vi "SCB-HMI.vi"() -> ()   [LabVIEW 2016]
uses:
  SC2 states.ctl
  Interface states.ctl
  Bypass control.ctl
  Minimum Times.ctl
  Vertical Rod states.ctl
  Horizontal Rod states.ctl
  GV states.ctl
panel:
  in  "Tab Control":T1(tab)
  in  "Start Rotate Wheel":bool
  in  "Wheel GV":bool
  in  "Ion Source GV":bool
  in  "Sample Rod":bool
  in  "Retract Rod":bool
  in  "Insert Rod":bool
  in  "Random Change":bool
  in  "Requested Sample":u8=32
  in  "Start Sample Change":bool
  in  "stop":bool
  out "Monitor state (CP)":T2=enum."Wait"
  out "Current Sample (CP)":u8
  out "Encoder Position":i32
  out "Converted Encoder":bool[](array[boolean])
  out "Raw Encoder":bool[](array[boolean])
  out "SCB State Control":T3=enum."wait"
  out "Current Sample":u8
  out "Change Complete?":bool
  out "Monitor State":T2=enum."Wait"
  out "Encoder Radius Readback":dbl=2.0
  out "Encoder Destination":i32
  out "Motor status":bool=TRUE
  out "Wheel GV Status":enum16{"status unclear", "closed", "open"}(ring)
  out "Insert Rod Status":enum16{"status unclear", "rod in", "rod out"}(ring)
  out "Ion Source GV Status":enum16{"status unclear", "closed", "open"}(ring)
  out "Sample Rod Status":enum16{"status unclear", "rod down", "rod up"}(ring)
  out "Retract Rod Status":enum16{"status unclear", "rod in", "rod out"}(ring)
  out "Sample Changer Status":string
  out "Requested Sample":u8
  in  "Bypass Cluster":T4
  in  "Encoder Radius":dbl=1.0
  in  "Encoder Offset":i16=-1021
  in  "Timeouts (ms)":T5={"Sample Rod"=10000, "Insert Rod"=10000, "Retract Rod"=10000, "Wheel GV"=10000, "Ion Source GV"=10000, "Rotate Wheel"=15000}
  in  "Minimum Times (ms)":T6={"Rotate Wheel Minimum Time"=1000}
  out "error out":errorcluster
  in  "error in (no error)":errorcluster
  # "Close"
  # "Open"
  # "Close"
  # "Open"
  # "Raise"
  # "Lower"
  # "Retract"
  # "Insert"
  # "Retract"
  # "Insert"
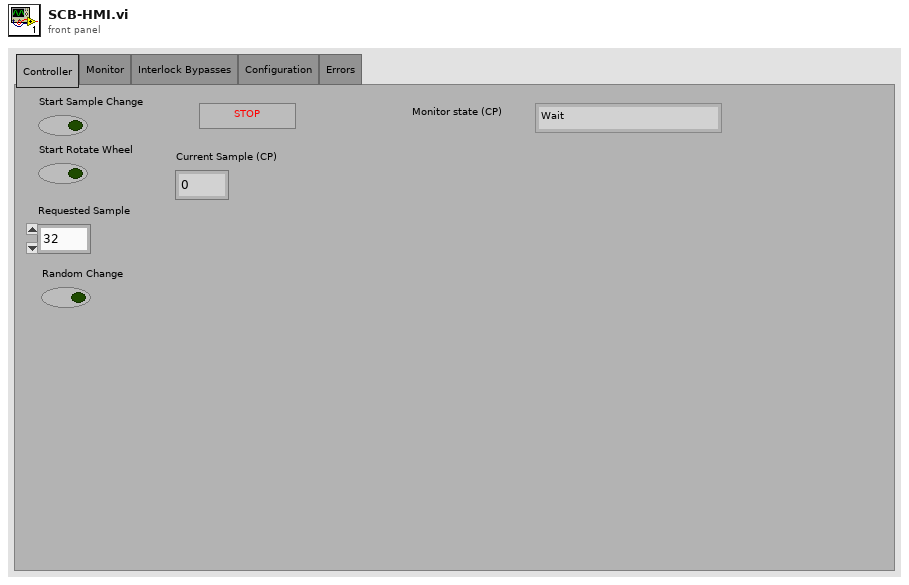
[diagram p1: front panel]
types:
  T1 = enum32{"Controller", "Monitor", "Interlock Bypasses", "Configuration", "Errors"}
  T2 = typedef "Interface states.ctl" = enum16{"Initialization", "Wait", "start wheel change", "Start Rotate Wheel", "Shutdown"}
  T3 = typedef "SC2 states.ctl" = enum16{"initialize", "wait", "change sample start", "change sample", "check position", "rotate wheel", "sample change complete", "sample rod up", "sample rod down", "retract rod in", "retract rod out", "insert rod in", "insert rod out", "wheel GV open", "wheel GV close", "ion source GV open", "ion source GV close", "vent source", "pump source", "Shutdown"}
  T4 = typedef "Bypass control.ctl" = cluster{"SCB Insert Rod Bypass":bool, "SCB Ion Source GV Bypass":bool, "SCB Retract Rod Bypass":bool, "SCB Sample Rod Bypass":bool, "SCB Wheel GV Bypass":bool}
  T5 = cluster{"Sample Rod":u16, "Insert Rod":u16, "Retract Rod":u16, "Wheel GV":u16, "Ion Source GV":u16, "Rotate Wheel":u16}
  T6 = typedef "Minimum Times.ctl" = cluster{"Rotate Wheel Minimum Time":u16}
  T7 = typedef "Horizontal Rod states.ctl" = enum16{"status unclear", "rod in", "rod out"}
  T8 = typedef "Vertical Rod states.ctl" = enum16{"status unclear", "rod down", "rod up"}
  T9 = typedef "GV states.ctl" = enum16{"status unclear", "closed", "open"}
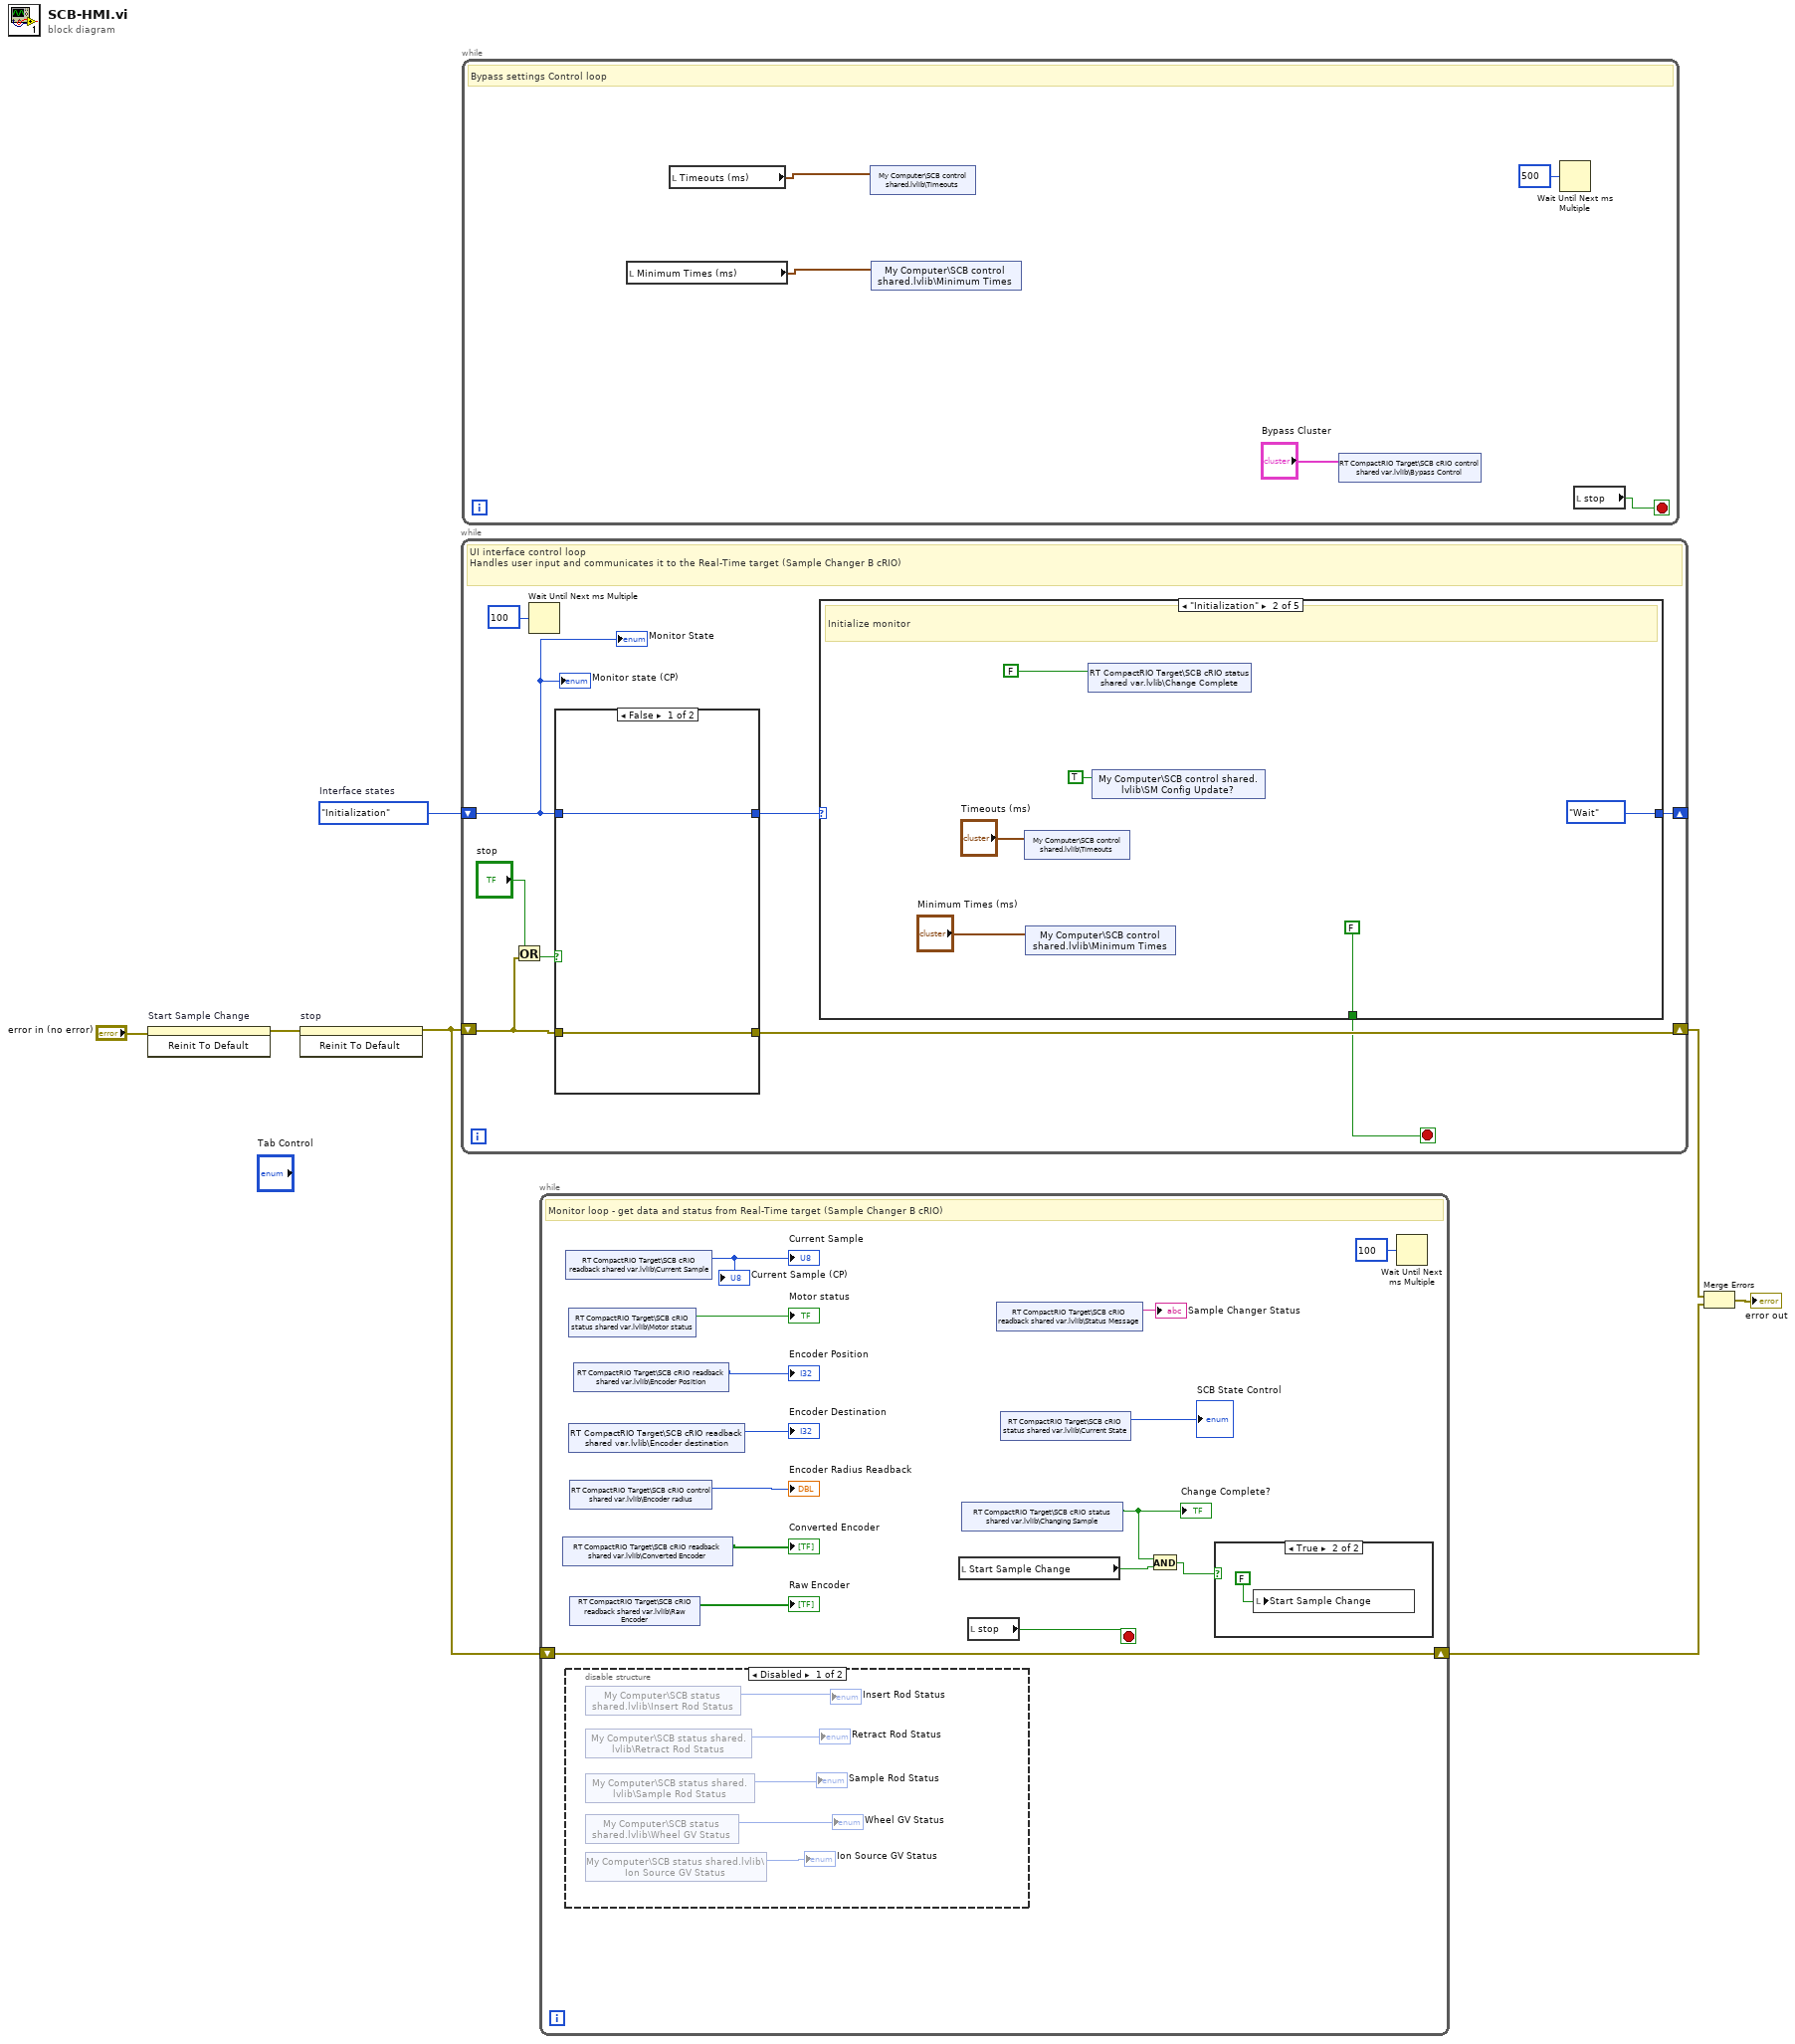
[diagram p0: block diagram]
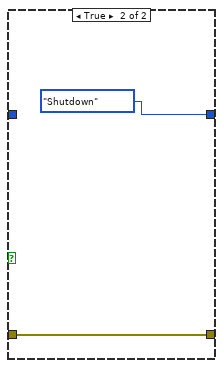
[diagram p4: hidden frame]
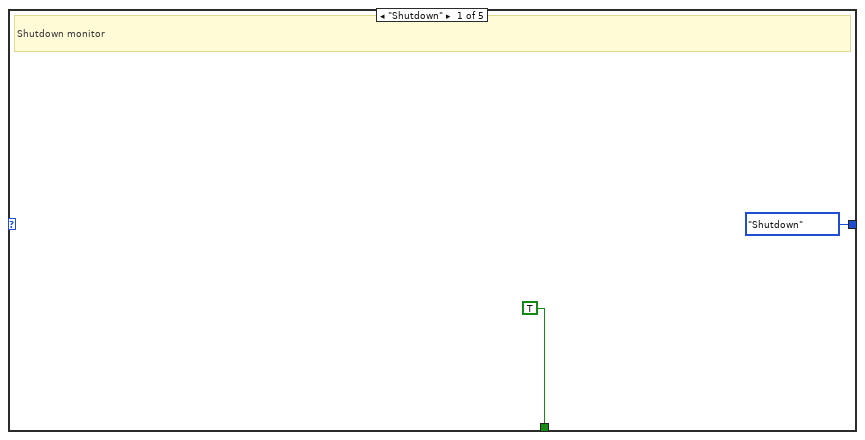
[diagram p5: hidden frame]
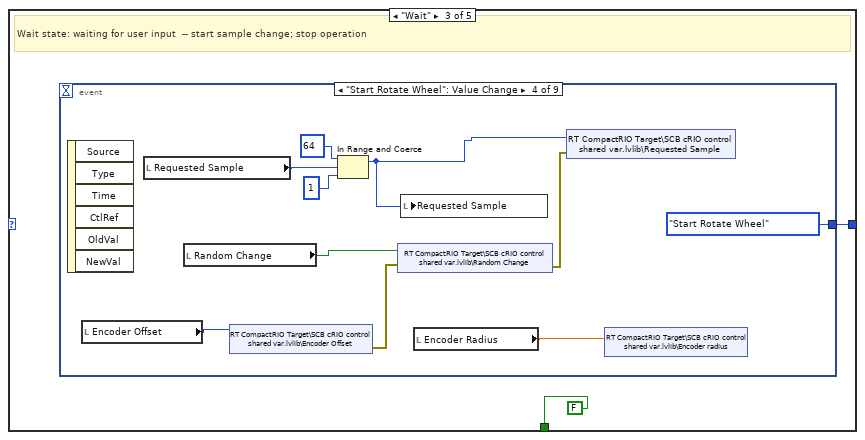
[diagram p6: hidden frame]
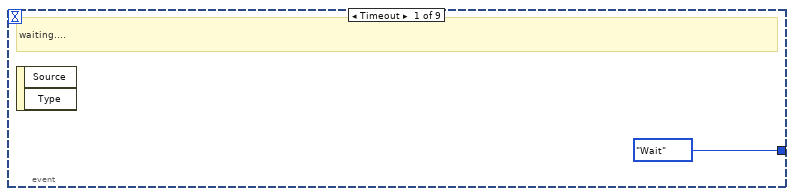
[diagram p7: hidden frame]
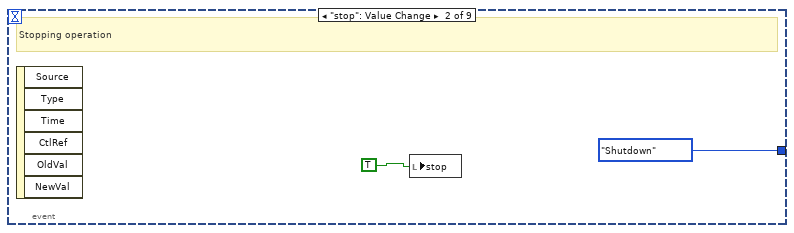
[diagram p8: hidden frame]
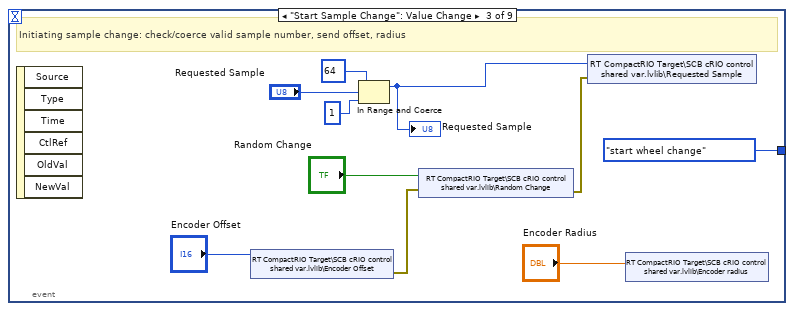
[diagram p9: hidden frame]
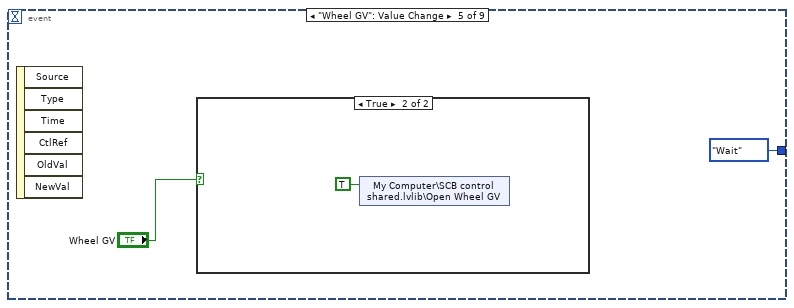
[diagram p10: hidden frame]
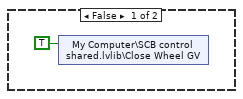
[diagram p11: hidden frame]
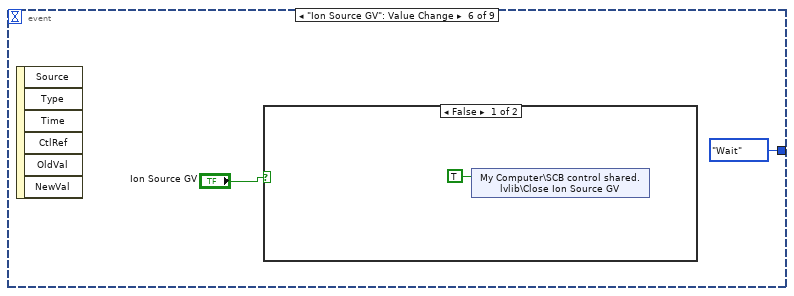
[diagram p12: hidden frame]
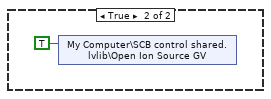
[diagram p13: hidden frame]
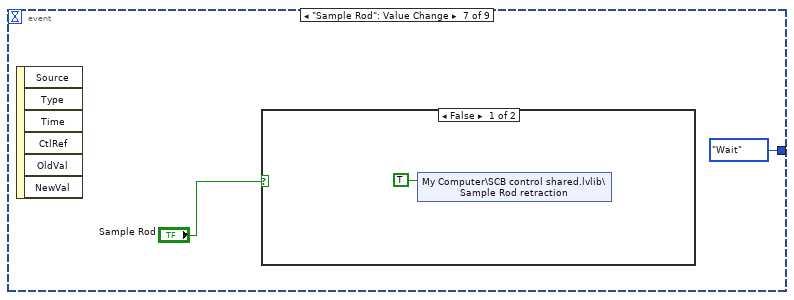
[diagram p14: hidden frame]
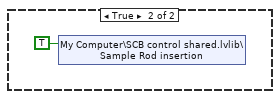
[diagram p15: hidden frame]
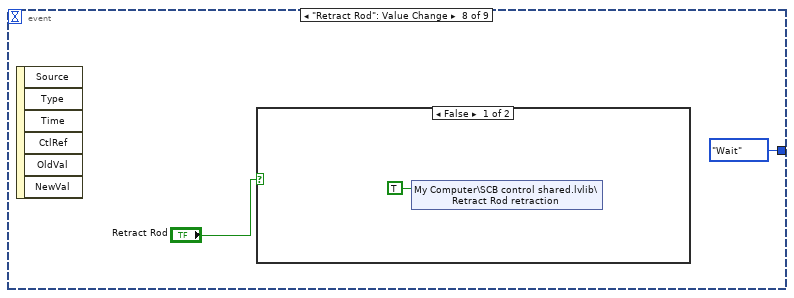
[diagram p16: hidden frame]
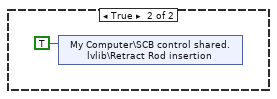
[diagram p17: hidden frame]
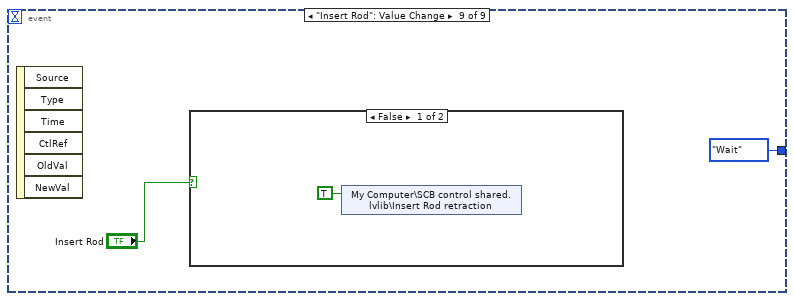
[diagram p18: hidden frame]
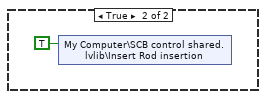
[diagram p19: hidden frame]
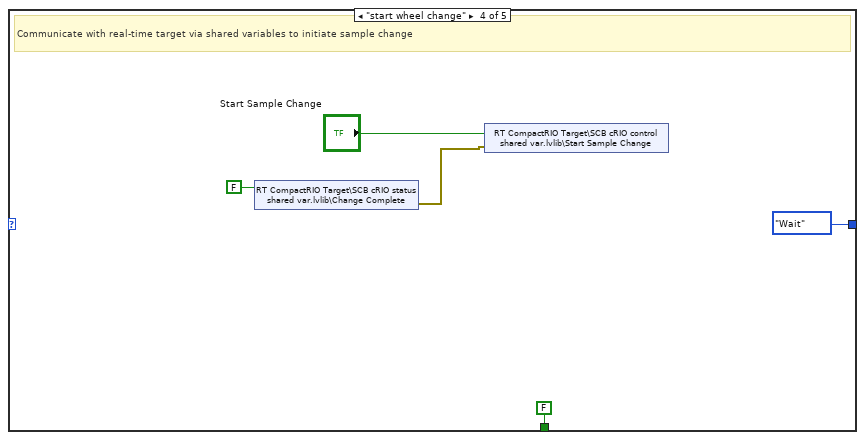
[diagram p20: hidden frame]
diagram:
  w4 = Interface_states."Initialization"  # Interface states
  n1 = invoke on="Start Sample Change" class="Bool (strict)" method="Reinit To Default"(error in="error in (no error)") -> (error out=w2:errorcluster)  [unwired: 2 in, 2 out]
  n2 = invoke on="stop" class="Bool (strict)" method="Reinit To Default"(error in=w2) -> (error out=w3:errorcluster)  [unwired: 2 in, 2 out]
  n3 = while {
    shift-right: [w13] -> w5
    shift-left: w3 -> [w9]
    shift-right: [w15] -> _
    shift-left: w4 -> [w11]
    stop <- w8 stop-if-true
    # "UI interface control loop\nHandles user input and communicates it to the Real-Time target (Sample Changer B cRIO)"
    n4 = Or(x="stop", y=w9) -> (x .or. y?=w10:bool)
    n5 = Wait Until Next ms Multiple(millisecond multiple=u32 100) -> ()  [unwired: 1 out]
    n6 = case shown="False" w10 {
      tunnel: w9 -> [w18 w19]
      tunnel: [w18 w19] -> w13
      tunnel: [w17 Interface_states."Shutdown" ("Interface states")] -> w12
      tunnel: w11 -> [w17 _]
      frame False {
      }
      frame True {
      }
    }
    n7 = case shown="\"Initialization\"" w12 {
      tunnel: [Interface_states."Shutdown" ("Interface states") Interface_states."Wait" ("Interface states") w29 Interface_states."Wait" ("Interface states") Interface_states."Wait" ("Interface states")] -> w15
      tunnel: [TRUE FALSE FALSE FALSE _] -> w8
      frame "Shutdown" {
        # "Shutdown monitor"
      }
      frame "Initialization" {
        # "Initialize monitor"
        n8 = shared-variable "My Computer\\SCB control shared.lvlib\\Timeouts"("Timeouts (ms)") -> ()  [unwired: 1 in, 1 out]
        n9 = shared-variable "My Computer\\SCB control shared.lvlib\\Minimum Times"("Minimum Times (ms)") -> ()  [unwired: 1 in, 1 out]
        n10 = shared-variable "RT CompactRIO Target\\SCB cRIO status shared var.lvlib\\Change Complete"(FALSE ("SC2 Change Complete")) -> ()  [unwired: 1 in, 1 out]
        n11 = shared-variable "My Computer\\SCB control shared.lvlib\\SM Config Update?"(TRUE ("SM Config Update?")) -> ()  [unwired: 1 in, 1 out]
      }
      frame "Wait" {
        # "Wait state: waiting for user input  -- start sample change; stop operation"
        n12 = event shown="[3] \"Start Rotate Wheel\": Value Change" {
          selector: _ -> [_ _ _ _ _ _ _ _ _]
          dyn-events: _ -> [_ _ _ _ _ _ _ _ _]
          timeout: _ -> [_ _ _ _ _ _ _ _ _]
          tunnel: [Interface_states."Wait" ("Interface states") Interface_states."Shutdown" ("Interface states") Interface_states."start wheel change" ("Interface states") Interface_states."Start Rotate Wheel" ("Interface states") Interface_states."Wait" ("Interface states") Interface_states."Wait" ("Interface states") Interface_states."Wait" ("Interface states") Interface_states."Wait" ("Interface states") Interface_states."Wait" ("Interface states")] -> w29
          event Timeout {
            # "waiting...."
            n13 = event-data() -> ()  [unwired: 1 in, 2 out]
          }
          event "stop": Value Change {
            # "Stopping operation"
            n14 = event-data() -> ()  [unwired: 1 in, 6 out]
            n15 = local write "stop"(TRUE ("stop")) -> ()
          }
          event "Start Sample Change": Value Change {
            # "Initiating sample change: check/coerce valid sample number, send offset, radius"
            n16 = event-data() -> ()  [unwired: 1 in, 6 out]
            n17 = shared-variable "RT CompactRIO Target\\SCB cRIO control shared var.lvlib\\Encoder Offset"("Encoder Offset") -> (error out=w37:errorcluster)  [unwired: 1 in]
            n18 = In Range and Coerce(upper limit=u8 64, x="Requested Sample", lower limit=u8 1) -> (coerced(x)=w39:u8)  [unwired: 1 out]
            "Requested Sample" <- w39
            n19 = shared-variable "RT CompactRIO Target\\SCB cRIO control shared var.lvlib\\Random Change"("Random Change", error in=w37) -> (error out=w38:errorcluster)
            n20 = shared-variable "RT CompactRIO Target\\SCB cRIO control shared var.lvlib\\Requested Sample"(w39, error in=w38) -> ()  [unwired: 1 out]
            n21 = shared-variable "RT CompactRIO Target\\SCB cRIO control shared var.lvlib\\Encoder radius"("Encoder Radius") -> ()  [unwired: 1 in, 1 out]
          }
          event "Start Rotate Wheel": Value Change {
            n22 = event-data() -> ()  [unwired: 1 in, 6 out]
            n23 = local read "Encoder Offset"() -> (w46:i16)
            n24 = local read "Requested Sample"() -> (w48:u8)
            n25 = local read "Random Change"() -> (w47:bool)
            n26 = shared-variable "RT CompactRIO Target\\SCB cRIO control shared var.lvlib\\Encoder Offset"(w46) -> (error out=w50:errorcluster)  [unwired: 1 in]
            n27 = In Range and Coerce(upper limit=u8 64, x=w48, lower limit=u8 1) -> (coerced(x)=w49:u8)  [unwired: 1 out]
            n28 = shared-variable "RT CompactRIO Target\\SCB cRIO control shared var.lvlib\\Random Change"(w47, error in=w50) -> (error out=w51:errorcluster)
            n29 = local write "Requested Sample"(w49) -> ()
            n30 = local read "Encoder Radius"() -> (w45:dbl)
            n31 = shared-variable "RT CompactRIO Target\\SCB cRIO control shared var.lvlib\\Requested Sample"(w49, error in=w51) -> ()  [unwired: 1 out]
            n32 = shared-variable "RT CompactRIO Target\\SCB cRIO control shared var.lvlib\\Encoder radius"(w45) -> ()  [unwired: 1 in, 1 out]
          }
          event "Wheel GV": Value Change {
            n33 = event-data() -> ()  [unwired: 1 in, 6 out]
            n34 = case shown="True" "Wheel GV" {
              frame False {
                n35 = shared-variable "My Computer\\SCB control shared.lvlib\\Close Wheel GV"(TRUE ("Close Wheel GV")) -> ()  [unwired: 1 in, 1 out]
              }
              frame True {
                n36 = shared-variable "My Computer\\SCB control shared.lvlib\\Open Wheel GV"(TRUE ("Open Wheel GV")) -> ()  [unwired: 1 in, 1 out]
              }
            }
          }
          event "Ion Source GV": Value Change {
            n37 = event-data() -> ()  [unwired: 1 in, 6 out]
            n38 = case shown="False" "Ion Source GV" {
              frame False {
                n39 = shared-variable "My Computer\\SCB control shared.lvlib\\Close Ion Source GV"(TRUE ("Close Ion Source GV")) -> ()  [unwired: 1 in, 1 out]
              }
              frame True {
                n40 = shared-variable "My Computer\\SCB control shared.lvlib\\Open Ion Source GV"(TRUE ("Open Ion Source GV")) -> ()  [unwired: 1 in, 1 out]
              }
            }
          }
          event "Sample Rod": Value Change {
            n41 = event-data() -> ()  [unwired: 1 in, 6 out]
            n42 = case shown="False" "Sample Rod" {
              frame False {
                n43 = shared-variable "My Computer\\SCB control shared.lvlib\\Sample Rod retraction"(TRUE ("Sample Rod retraction")) -> ()  [unwired: 1 in, 1 out]
              }
              frame True {
                n44 = shared-variable "My Computer\\SCB control shared.lvlib\\Sample Rod insertion"(TRUE ("Sample Rod insertion")) -> ()  [unwired: 1 in, 1 out]
              }
            }
          }
          event "Retract Rod": Value Change {
            n45 = event-data() -> ()  [unwired: 1 in, 6 out]
            n46 = case shown="False" "Retract Rod" {
              frame False {
                n47 = shared-variable "My Computer\\SCB control shared.lvlib\\Retract Rod retraction"(TRUE ("Retract Rod retraction")) -> ()  [unwired: 1 in, 1 out]
              }
              frame True {
                n48 = shared-variable "My Computer\\SCB control shared.lvlib\\Retract Rod insertion"(TRUE ("Retract Rod insertion")) -> ()  [unwired: 1 in, 1 out]
              }
            }
          }
          event "Insert Rod": Value Change {
            n49 = event-data() -> ()  [unwired: 1 in, 6 out]
            n50 = case shown="False" "Insert Rod" {
              frame False {
                n51 = shared-variable "My Computer\\SCB control shared.lvlib\\Insert Rod retraction"(TRUE ("Insert Rod retraction")) -> ()  [unwired: 1 in, 1 out]
              }
              frame True {
                n52 = shared-variable "My Computer\\SCB control shared.lvlib\\Insert Rod insertion"(TRUE ("Insert Rod insertion")) -> ()  [unwired: 1 in, 1 out]
              }
            }
          }
        }
      }
      frame "start wheel change" {
        # "Communicate with real-time target via shared variables to initiate sample change"
        n53 = shared-variable "RT CompactRIO Target\\SCB cRIO status shared var.lvlib\\Change Complete"(FALSE ("SC2 Change Complete")) -> (error out=w74:errorcluster)  [unwired: 1 in]
        n54 = shared-variable "RT CompactRIO Target\\SCB cRIO control shared var.lvlib\\Start Sample Change"("Start Sample Change", error in=w74) -> ()  [unwired: 1 out]
      }
      frame "Start Rotate Wheel" {
        n55 = shared-variable "My Computer\\SCB control shared.lvlib\\Rotate Wheel"("Start Rotate Wheel") -> ()  [unwired: 1 in, 1 out]
      }
    }
    "Monitor State" <- w11
    "Monitor state (CP)" <- w11
  }
  n56 = while {
    stop <- w84 stop-if-true
    # "Bypass settings Control loop"
    n57 = local read "Minimum Times (ms)"() -> (w81:T6)
    n58 = local read "Timeouts (ms)"() -> (w82:T5)
    n59 = shared-variable "My Computer\\SCB control shared.lvlib\\Timeouts"(w82) -> ()  [unwired: 1 in, 1 out]
    n60 = shared-variable "My Computer\\SCB control shared.lvlib\\Minimum Times"(w81) -> ()  [unwired: 1 in, 1 out]
    n61 = shared-variable "RT CompactRIO Target\\SCB cRIO control shared var.lvlib\\Bypass Control"("Bypass Cluster") -> ()  [unwired: 1 in, 1 out]
    n62 = Wait Until Next ms Multiple(millisecond multiple=u32 500) -> ()  [unwired: 1 out]
    n63 = local read "stop"() -> (w84:bool)
  }
  n64 = while {
    shift-right: [w99] -> w6
    shift-left: w3 -> [w99]
    stop <- w98 stop-if-true
    # "Monitor loop - get data and status from Real-Time target (Sample Changer B cRIO)"
    n65 = shared-variable "RT CompactRIO Target\\SCB cRIO readback shared var.lvlib\\Converted Encoder"() -> (→"Converted Encoder":bool[])  [unwired: 1 in, 1 out]
    n66 = shared-variable "RT CompactRIO Target\\SCB cRIO readback shared var.lvlib\\Current Sample"() -> (→"Current Sample" →"Current Sample (CP)":u8)  [unwired: 1 in, 1 out]
    n67 = disable-structure shown="Disabled" {
      frame Disabled {
        n68 = shared-variable "My Computer\\SCB status shared.lvlib\\Insert Rod Status"() -> (→"Insert Rod Status":T7)  [unwired: 1 in, 1 out]
        n69 = shared-variable "My Computer\\SCB status shared.lvlib\\Retract Rod Status"() -> (→"Retract Rod Status":T7)  [unwired: 1 in, 1 out]
        n70 = shared-variable "My Computer\\SCB status shared.lvlib\\Sample Rod Status"() -> (→"Sample Rod Status":T8)  [unwired: 1 in, 1 out]
        n71 = shared-variable "My Computer\\SCB status shared.lvlib\\Wheel GV Status"() -> (→"Wheel GV Status":T9)  [unwired: 1 in, 1 out]
        n72 = shared-variable "My Computer\\SCB status shared.lvlib\\Ion Source GV Status"() -> (→"Ion Source GV Status":T9)  [unwired: 1 in, 1 out]
      }
      frame Enabled {
      }
    }
    n73 = shared-variable "RT CompactRIO Target\\SCB cRIO status shared var.lvlib\\Motor status"() -> (→"Motor status":bool)  [unwired: 1 in, 1 out]
    n74 = shared-variable "RT CompactRIO Target\\SCB cRIO readback shared var.lvlib\\Encoder destination"() -> (→"Encoder Destination":i32)  [unwired: 1 in, 1 out]
    n75 = shared-variable "RT CompactRIO Target\\SCB cRIO control shared var.lvlib\\Encoder radius"() -> (→"Encoder Radius Readback":i32)  [unwired: 1 in, 1 out]
    n76 = shared-variable "RT CompactRIO Target\\SCB cRIO readback shared var.lvlib\\Raw Encoder"() -> (→"Raw Encoder":bool[])  [unwired: 1 in, 1 out]
    n77 = shared-variable "RT CompactRIO Target\\SCB cRIO readback shared var.lvlib\\Encoder Position"() -> (→"Encoder Position":i32)  [unwired: 1 in, 1 out]
    n78 = local read "Start Sample Change"() -> (w96:bool)
    n79 = shared-variable "RT CompactRIO Target\\SCB cRIO status shared var.lvlib\\Changing Sample"() -> (w94:bool)  [unwired: 1 in, 1 out]
    "Change Complete?" <- w94
    n80 = local read "stop"() -> (w98:bool)
    n81 = shared-variable "RT CompactRIO Target\\SCB cRIO readback shared var.lvlib\\Status Message"() -> (→"Sample Changer Status":string)  [unwired: 1 in, 1 out]
    n82 = shared-variable "RT CompactRIO Target\\SCB cRIO status shared var.lvlib\\Current State"() -> (→"SCB State Control":T3)  [unwired: 1 in, 1 out]
    n83 = And(x=w94, y=w96) -> (x .and. y?=w97:bool)
    n84 = case shown="True" w97 {
      frame False {
      }
      frame True {
        n85 = local write "Start Sample Change"(FALSE ("Start Sample Change")) -> ()
      }
    }
    n86 = Wait Until Next ms Multiple(millisecond multiple=u32 100) -> ()  [unwired: 1 out]
  }
  n87 = Merge Errors(w5, w6) -> (→"error out":errorcluster)
